vi "Auto-Gyro.vi"(5 "GyroDevRef":T1) -> (0 "Angle":dbl, 1 "X-Axis Out":dbl format="%.2f", 2 "GyroDevRef Out":T1)   [LabVIEW 2011]
uses:
  <vilib>/Rock Robotics/WPI/Gyro/WPI_GyroDevRef.ctl
  <vilib>/Rock Robotics/SystemInterfaces/Typedef/FPGA_TypedefAnalogModule.ctl
  <vilib>/Rock Robotics/SystemInterfaces/AI/FPGA_AIChannel.ctl
  <vilib>/addons/control/pid/pid.llb/PID (DBL).vi
  <vilib>/addons/control/pid/NI_PID_pid.lvlib
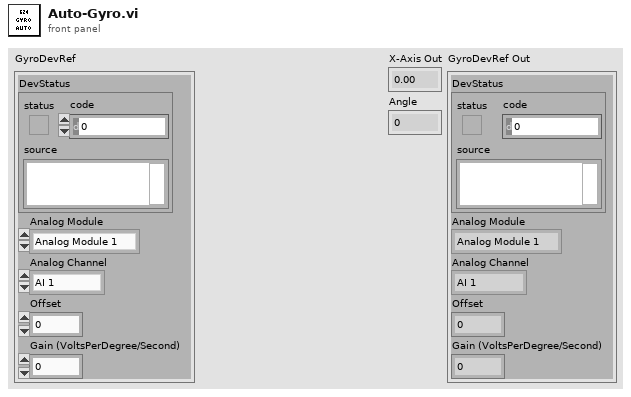
[diagram p1: front panel]
types:
  T1 = typedef "WPI_GyroDevRef.ctl" = cluster{"DevStatus":errorcluster, "Analog Module":T2, "Analog Channel":T3, "Offset":dbl, "Gain (VoltsPerDegree/Second)":dbl}
  T2 = typedef "FPGA_TypedefAnalogModule.ctl" = enum16{"Analog Module 1", "Analog Module 2"}
  T3 = typedef "FPGA_AIChannel.ctl" = enum8{"AI 1", "AI 2", "AI 3", "AI 4", "AI 5", "AI 6", "AI 7", "AI 8", "Invalid"}
  T4 = cluster{"proportional gain (Kc)":dbl, "integral time (Ti, min)":dbl, "derivative time (Td, min)":dbl}
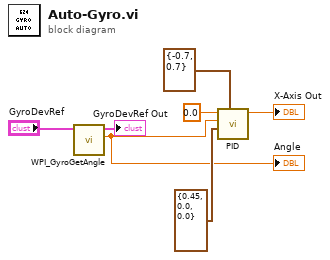
[diagram p0: block diagram]
diagram:
  n1 = call <vilib>:"WPI_GyroGetAngle.vi"("GyroDevRef"="GyroDevRef") -> ("Angle"=w4:dbl, "GyroDevRef"=→"GyroDevRef Out":T1)  [unwired: 7 in, 2 out]
  "Angle" <- w4
  n2 = call-poly <vilib>:"PID.vi"("output range"=cluster{"output high":dbl, "output low":dbl} {"output high"=-0.7, "output low"=0.7}, "PID gains"=T4 {"proportional gain (Kc)"=0.45, "integral time (Ti, min)"=0.0, "derivative time (Td, min)"=0.0}, "process variable"=w4, "setpoint"=0.0) -> ("output"=→"X-Axis Out":dbl)  [unwired: 6 in, 1 out]
